vi "LockToLS.vi"(8 "error in (no error)":errorcluster, 10 "LockToLS":T1, 11 "ChassisCfg":refnum<class "ChassisCfg.lvclass">) -> (0 "error out":errorcluster, 3 "ChassisCfg":refnum<class "ChassisCfg.lvclass">)   [LabVIEW 2012, in "Configuration Grandmaster.lvlib" / "ChassisCfg.lvclass"]
uses:
  ChassisCfg.lvclass
  Common/Controls/LS Lock Sizes.ctl
  ChassisCfg.lvclass/ChassisCfg.ctl
  Common/Controls/TE_Designator.ctl
  Class Timing Group/Read Rate.vi
  Class Timing Group/TimingGrp.lvclass
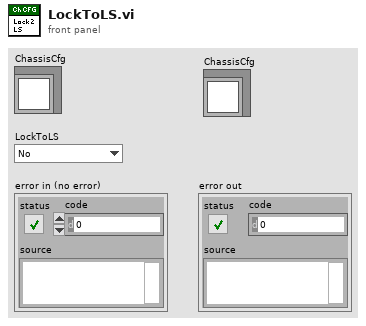
[diagram p1: front panel]
types:
  T1 = typedef "LS Lock Sizes.ctl" = enum16{"No", "250ms", "500ms", "1s"}
  T2 = typedef "TE_Designator.ctl" = enum16{"High Speed", "Low Speed"}
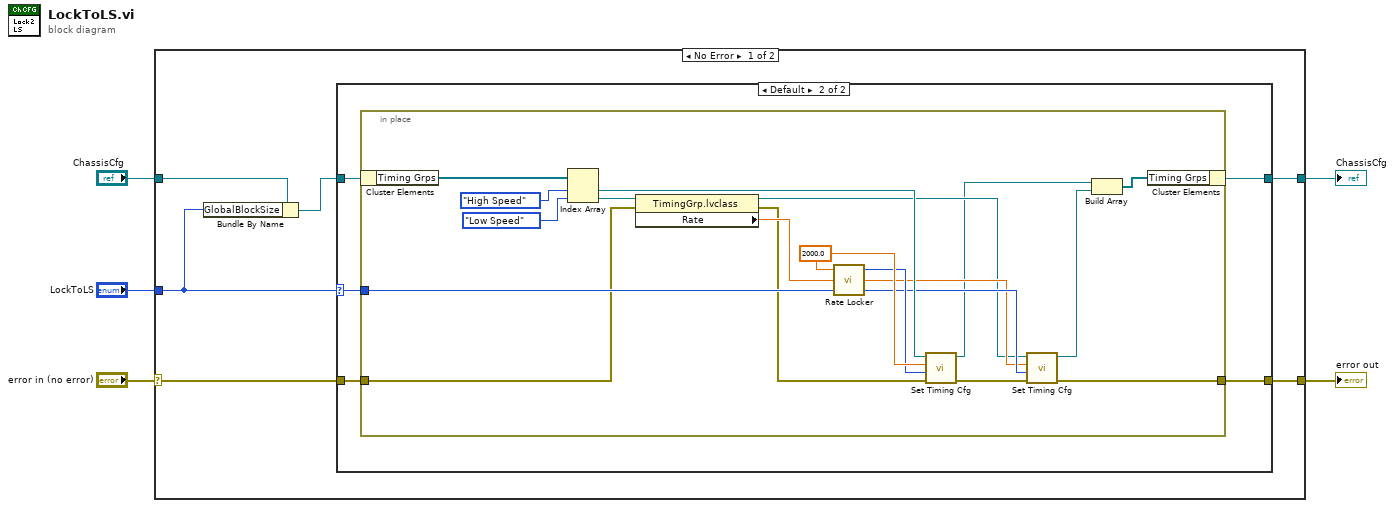
[diagram p0: block diagram]
diagram:
  n1 = case shown="No Error" "error in (no error)" {
    selector: "error in (no error)" -> [w6 w39]
    tunnel: [w11 w39] -> w5
    tunnel: [w10 w38] -> w4
    tunnel: "ChassisCfg" -> [w9 w38]
    tunnel: "LockToLS" -> [w7 _]
    frame No Error {
      n2 = Bundle By Name(cluster=w9, "GlobalBlockSize"=w7) -> (w8:refnum<class "ChassisCfg.lvclass">)
      n3 = case shown="Default" w7 {
        selector: w7 -> [_ w14]
        tunnel: [w12 w18] -> w11
        tunnel: w6 -> [w12 w17]
        tunnel: [w13 w16] -> w10
        tunnel: w8 -> [w13 w15]
        frame "No" {
        }
        frame Default {
          n4 = in-place {
            in-place-border: w14 -> [w31]
            in-place-border: [w19] -> w18
            in-place-border: w17 -> [w23]
            w30 = 2000.0 ("Config Grandmaster.GrpTiming.HSCfg.Rate")
            n5 = in-place-cluster #1(w15) -> ("Timing Grps"=w22:refnum<class "TimingGrp.lvclass">[])
            n6 = Index Array(array=w22, index #1=TE_Designator."High Speed" ("Timing Engine"), index #2=TE_Designator."Low Speed" ("Timing Engine")) -> (element #1=w37:refnum<class "TimingGrp.lvclass">, element #2=w36:refnum<class "TimingGrp.lvclass">)
            n7 = property class="TimingGrp.lvclass"(reference=w36, error in=w23) -> (reference out=w26:refnum<class "TimingGrp.lvclass">, error out=w24:errorcluster, "Rate"=w32:dbl)
            n8 = call "Rate Locker.vi"("LockToLS"=w31, "LSCfg.Rate"=w32, "HSCfg.Rate"=w30) -> ("LSCfg.ReadBlk"=w28:i32, "LSCfg.Rate"=w27:dbl, "HS Block Size"=w29:i32)
            n9 = call "Set Timing Cfg.vi"("error in"=w24, "ReadBlk"=w29, "Rate"=w30, "TimingGrp in"=w37) -> ("error out"=w25:errorcluster, "TimingGrp in"=w20:refnum<class "TimingGrp.lvclass">)  [unwired: 6 in]
            n10 = call "Set Timing Cfg.vi"("error in"=w25, "ReadBlk"=w28, "Rate"=w27, "TimingGrp in"=w26) -> ("error out"=w19:errorcluster, "TimingGrp in"=w35:refnum<class "TimingGrp.lvclass">)  [unwired: 6 in]
            n11 = Build Array(w20, w35) -> (w21:refnum<class "TimingGrp.lvclass">[])
            n12 = in-place-cluster #1("Timing Grps"=w21) -> (w16:refnum<class "ChassisCfg.lvclass">)
          }
        }
      }
    }
    frame Error {
    }
  }
  "ChassisCfg" <- w4
  "error out" <- w5
